vi "Hex array to character string.vi"(11 "Array":string[][](array[string])) -> (3 "String":string)   [LabVIEW 2020]
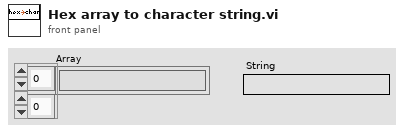
[diagram p1: front panel]
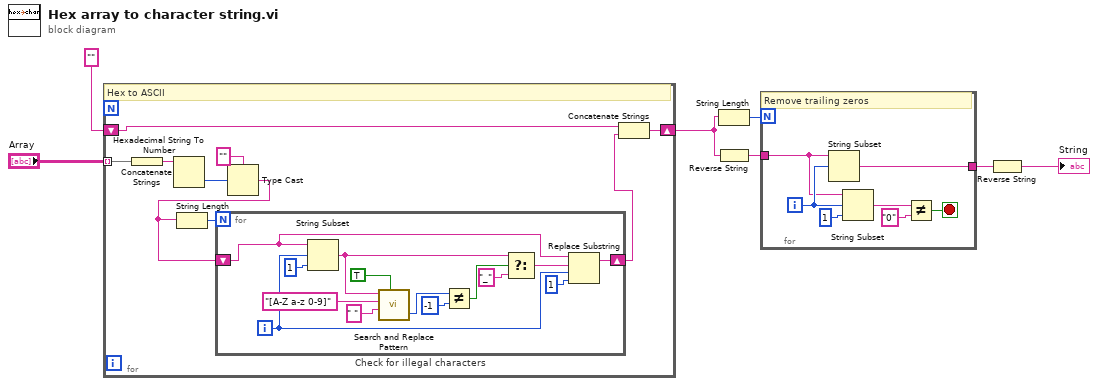
[diagram p0: block diagram]
diagram:
  n1 = for {
    tunnel: "Array" -> [w13] mode=indexing
    shift-right: [w14] -> w1
    shift-left: "" -> [w11]
    # "Hex to ASCII"
    n2 = Concatenate Strings(w13) -> (w12:string)
    n3 = Hexadecimal String To Number(string=w12) -> (number=w15:u32)  [unwired: 2 in, 1 out]
    n4 = Type Cast(type="", x=w15) -> (*(type *) &x=w9:string)
    n5 = String Length(string=w9) -> (length=w8:i32)
    n6 = for "Check for illegal characters" {
      N: w8 -> [_]
      shift-right: [w17] -> w10
      shift-left: w9 -> [w22]
      i -> [w20]
      n7 = String Subset(string=w22, offset (0)=w20, length (rest)=1 ("length (rest)")) -> (substring=w18:string)
      n8 = call <vilib>:"Search and Replace Pattern.vi"("string"=w18, "regular expression (\"\")"="[A-Z a-z 0-9]" ("regular expression (\"\")"), "replace string (\"\")"=" " ("replace string (\"\")"), "replace all? (F)"=TRUE) -> ("offset past match"=w26:i32)  [unwired: 1 in, 1 out]
      n9 = Not Equal?(x=w26, y=-1) -> (x != y?=w24:bool)
      n10 = Select(t=w18, s=w24, f="_") -> (s? t:f=w19:string)
      n11 = Replace Substring(2:1 ("length (len. of substring)"), 3:w20, 4:w19, 5:w22) -> (1:w17:string)  [unwired: 1 out]
    }
    n12 = Concatenate Strings(w11, w10) -> (w14:string)
  }
  n13 = String Length(string=w1) -> (length=w3:i32)
  n14 = Reverse String(1:w1) -> (0:w2:string)
  n15 = for {
    N: w3 -> [_]
    tunnel: w2 -> [w32]
    tunnel: [w35] -> w4
    i -> [w34]
    stop <- w36 stop-if-true
    # "Remove trailing zeros"
    n16 = String Subset(string=w32, offset (0)=w34) -> (substring=w35:string)  [unwired: 1 in]
    n17 = String Subset(string=w32, offset (0)=w34, length (rest)=1 ("length (rest)")) -> (substring=w31:string)
    n18 = Not Equal?(x=w31, y="0") -> (x != y?=w36:bool)
  }
  n19 = Reverse String(1:w4) -> (0:→"String":string)
